vi "robotmodes.vi"() -> ()   [LabVIEW 2018]
panel:
  out "Auto_Subsystem_Action":path
  out "Auto_Drive_Action":string
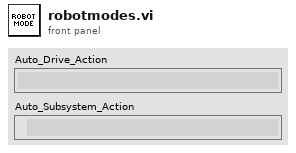
[diagram p1: front panel]
diagram:
